vi "Fit.vi"(8 "error in (no error)":errorcluster caption="entrée d'erreur (pas d'erreur)", 9 "y":string[][](array[string]), 10 "X":string[][](array[string]), 11 "Nystroem.lvclass":refnum<class "Nystroem.lvclass">) -> (0 "error out":errorcluster caption="sortie d'erreur", 2 "String Data":string, 3 "Nystroem.lvclass":refnum<class "Nystroem.lvclass">)   [LabVIEW 2020, in "Nystroem.lvclass"]
doc: "Fit estimator to data.\n\nSamples a subset of training points, computes kernel on these and computes normalization matrix.\n\nReturns : \n\n- String : OK"
uses:
  Nystroem.lvclass
  Nystroem.lvclass/Nystroem.ctl
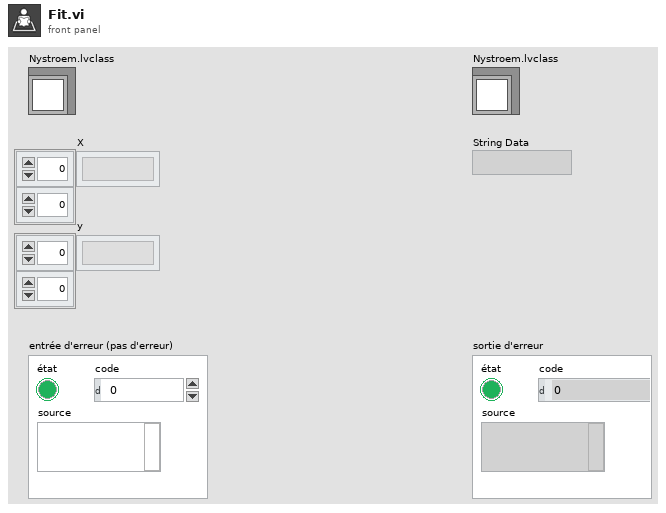
[diagram p1: front panel]
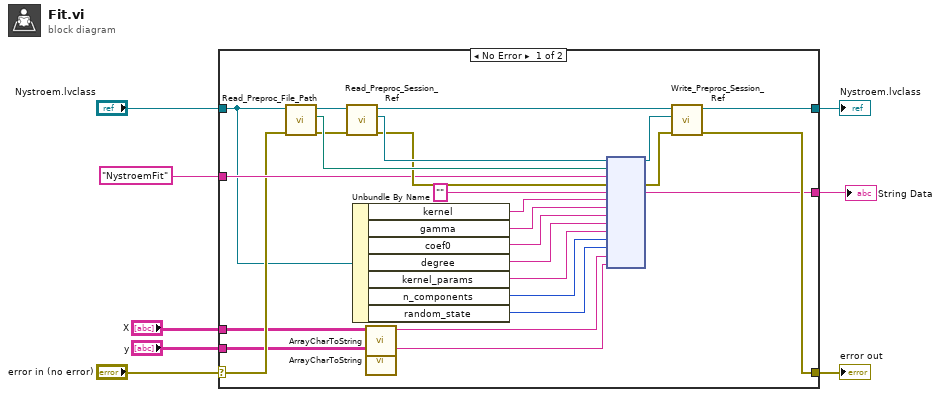
[diagram p0: block diagram]
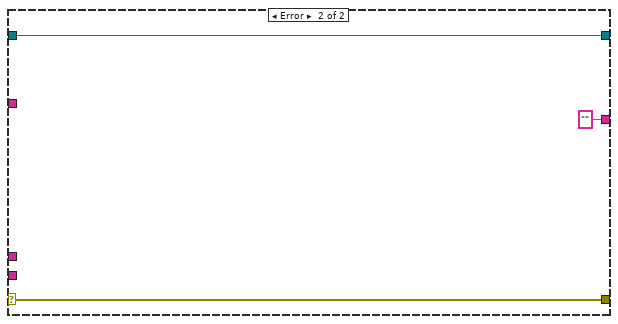
[diagram p2: hidden frame]
diagram:
  n1 = case shown="No Error" "error in (no error)" {
    selector: "error in (no error)" -> [w22 w37]
    tunnel: [w20 w37] -> w7
    tunnel: [w9 w36] -> w5
    tunnel: "Nystroem.lvclass" -> [w21 w36]
    tunnel: "NystroemFit" ("Fonction") -> [w23 _]
    tunnel: "X" -> [w13 _]
    tunnel: [w14 ""] -> w2
    tunnel: "y" -> [w11 _]
    frame No Error {
      n2 = call-dynamic "Read_Preproc_File_Path.vi"("error in (no error)"=w22, "Python in"=w21) -> ("error out"=w29:errorcluster, "File_Path"=w32:path, "Python out"=w34:refnum<class "Nystroem.lvclass">)  [unwired: 7 in]
      n3 = call-dynamic "Read_Preproc_Session_Ref.vi"("error in (no error)"=w29, "Python in"=w34) -> ("error out"=w30:errorcluster, "Session_ref"=w31:refnum<k35>, "Python out"=w33:refnum<class "Nystroem.lvclass">)  [unwired: 7 in]
      n4 = Unbundle By Name(w21) -> ("kernel"=w25:string, "gamma"=w24:string, "coef0"=w19:string, "degree"=w18:string, "kernel_params"=w17:string, "n_components"=w16:i32, "random_state"=w15:i32)
      n5 = call "ArrayCharToString.vi"("TAB"=w13) -> ("Instruction"=w12:string)  [unwired: 10 in]
      n6 = call "ArrayCharToString.vi"("TAB"=w11) -> ("Instruction"=w10:string)  [unwired: 10 in]
      n7 = node(w31, w32, w23, w30, "", w25, w24, w19, w18, w17, w16, w15, w12, w10) -> (w26:refnum<k35>, w28:errorcluster, w14:string)  [unwired: 9 in, 2 out]
      n8 = call-dynamic "Write_Preproc_Session_Ref.vi"("error in (no error)"=w28, "Session_ref"=w26, "Python in"=w33) -> ("error out"=w20:errorcluster, "Python out"=w9:refnum<class "Nystroem.lvclass">)  [unwired: 7 in]
    }
    frame Error {
    }
  }
  "error out" <- w7
  "Nystroem.lvclass" <- w5
  "String Data" <- w2
